vi "Motion.vi"(8 "error in (no error)":errorcluster, 10 "Controle":T1, 11 "map reference in":refnum<data-value>) -> (0 "error out":errorcluster, 2 "Indicator":T1, 3 "map reference out":refnum<data-value>)   [LabVIEW 2012]
uses:
  <vilib>/robotics/Navigation/shared/WorldMap/OccupancyGridWorldMap/NI_Robotics_OccupancyGridWorldMap.lvclass
  Utilities/Robot Parameters/Robot Parameters.vi
panel:
  in  "Delta X":i32
  in  "Delta Y":i32
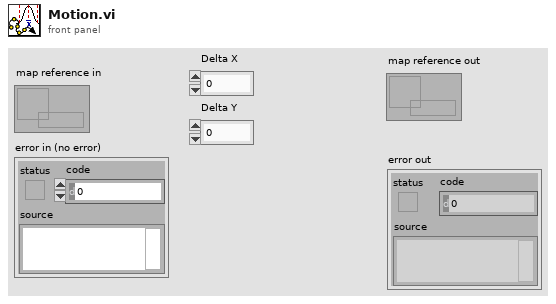
[diagram p1: front panel]
types:
  T1 = cluster{"Resolution":i32, "Scale":dbl, "Data":cluster{"GPS Data":cluster{"Latitude":dbl, "Longitude":dbl, "Altitude":dbl, "Velocity, Correction & SET":cluster{"Velocity North":dbl, "Velocity East":dbl, "Velocity Up":dbl, "Ellipsoidal Height":dbl, "GDOP":sgl, "PDOP":sgl, "HDOP":sgl, "VDOP":sgl, "TDOP":sgl, "Horizontal Figure of Merit":u8, "Time Figure of Merit":u8, "Max dGPS Age":sgl, "Extended Navigation Mode":u8, "Antenna Height Adjustment ":dbl, "SET North":i32, "SET East":i32, "SET Up":i32}, "Time":cluster{"GPS Week":u16, "GPS Time of Week":sgl}, "Satellites Used":i32[]}, "IMU Data":cluster{"Position":cluster{"Roll":dbl, "Pitch":dbl, "Yaw":dbl}, "Orientation Matrix":dbl[][], "Magnetic Field":cluster{"Z-Axis Magnetic Field":dbl, "Y-Axis Magnetic Field":dbl, "X-Axis Magnetic Field":dbl}, "Acceleration":cluster{"Z-Axis Acceleration":dbl, "Y-Axis Acceleration":dbl, "X-Axis Acceleration":dbl}, "Angular Rate":cluster{"X-Axis Angular Rate":dbl, "Y-Axis Angular Rate":dbl, "Z-Axis Angular Rate":dbl}, "Quaternion":dbl[]}, "LIDAR Data":cluster{"Magnitude":dbl[], "Direction":dbl[]}, "Telemetry":cluster{"Voltage":cluster{sgl, sgl, sgl}, "Encoder Speed":cluster{i32, i32}, "Temps":cluster{"IC Temp (C)":i32, "Ch1 Temp (C)":i32, "Ch2 Temp (C)":i32}, "Current":cluster{dbl, dbl, dbl, dbl}}, "Lines":cluster{"Start Point":cluster{"X":sgl, "Y":sgl}, "End Point":cluster{"X":sgl, "Y":sgl}, "Length":dbl, "Orientation":dbl, "Score":dbl}[]}, "initialized array":dbl[][]}
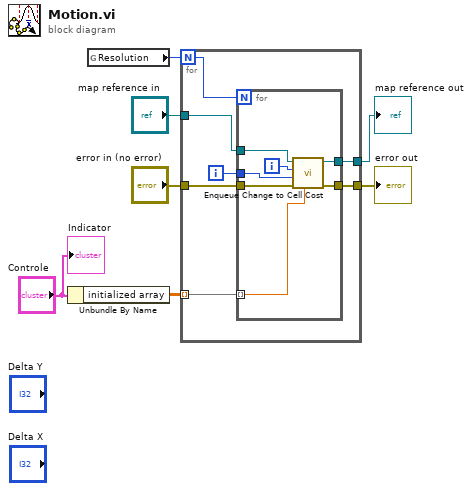
[diagram p0: block diagram]
diagram:
  n1 = Unbundle By Name("Controle") -> ("initialized array"=w1:dbl[][])
  n2 = global read "Robot Parameters.vi" "Resolution"() -> (w3:i32)
  n3 = for {
    N: w3 -> [w9]
    tunnel: "map reference in" -> [w14]
    tunnel: [w13] -> w4
    tunnel: "error in (no error)" -> [w11]
    tunnel: [w10] -> w5
    tunnel: w1 -> [w8] mode=indexing
    i -> [w12]
    n4 = for {
      N: w9 -> [_]
      tunnel: w14 -> [w21]
      tunnel: [w20] -> w13
      tunnel: w12 -> [w18]
      tunnel: w11 -> [w17]
      tunnel: [w16] -> w10
      tunnel: w8 -> [w15] mode=indexing
      i -> [w19]
      n5 = call <vilib>:"Enqueue Change to Cell Cost.vi"("cost"=w15, "error in (no error)"=w17, "y"=w18, "x"=w19, "map reference in"=w21) -> ("error out"=w16:errorcluster, "map reference out"=w20:refnum<data-value>)  [unwired: 5 in]
    }
  }
  "map reference out" <- w4
  "error out" <- w5
  "Indicator" <- "Controle"
